vi "FRIC_navX_Internal_SPI_ProcessingLoop.vi"(7 "Device Number":T2, 11 "Rate (4Hz-200Hz)":u8=50 min=4 max=200) -> ()   [LabVIEW 2016]
doc: "This navX VI handles the reading/writing for the navX. All of the good stuff is in here.\nTHIS VI SHOULD NOT BE CALLED BY THE USER!"
uses:
  <vilib>/Rock Robotics/SystemInterfaces/spilib/spi_bus.ctl
  _TypeDefs/FRIC_navX_DeviceNumbersTypeDef.ctl
  _TypeDefs/FRIC_navX_I2C Process Loop TypeDef.ctl
  _TypeDefs/FRIC_navX_ProcessingLoopStatesTypeDef_I2C.ctl
  _TypeDefs/Z900_navX_DeviceTypeDef.ctl
  _TypeDefs/Z900_navX_ProtocolTypeDef.ctl
  _TypeDefs/Z900_navX_NotifyPacketTypeDef.ctl
  _TypeDefs/Z900_navX_ActionTypeDef.ctl
  _TypeDefs/Z900_navX_SerialStreamTypeDef.ctl
  <vilib>/Rock Robotics/SystemInterfaces/i2clib/i2c_bus.ctl
  _TypeDefs/Z900_navX_IntegrationControlRegisters.ctl
  <vilib>/Rock Robotics/WPI/SPI/WPI_SPIDevRef.ctl
  <vilib>/Rock Robotics/WPI/SerialPort/WPI_SerialPort.ctl
  <vilib>/Rock Robotics/WPI/SerialPort/WPI_SerialPortRef.ctl
  <vilib>/Platform/TimedLoop/XDataNode/timing_clust.ctl
  <vilib>/Platform/TimedLoop/XDataNode/nitl_modes.ctl
  <vilib>/Platform/TimedLoop/XDataNode/wakeup.ctl
  _TypeDefs/Flags/Z900_navX_Flags_CapabilityTypeDef.ctl
  _TypeDefs/Z900_navX_DeviceRegisters.ctl
  _Util/Z900_navX_Util_LittleEndian_to_BigEndian.vi
  <vilib>/Rock Robotics/SystemInterfaces/Utilities/FPGA_UtilitiesRead LocalTime.vi
  <vilib>/Platform/TimedLoop/XDataNode/XDataNode.xnode
  <vilib>/Platform/TimedLoop/XDataNode/XDNodeRunTimeDep.lvlib
  <vilib>/ptbypt/NI_PtbyPt.lvlib
panel:
  in  "Tab Control":enum32{"Page 1", "Page 2"}(tab)
  in  "Halt":bool
  out "Connected":bool
  in  "SPI Bus":T1=enum."SPI MXP"
  in  "Clock Rate (Hz)":dbl=2000000.0 format="%_6f"
  out "error":errorcluster
  out "Delay":dbl
  out "Loop Time":dbl format="%0.2f"
  out "Loop dt":i64
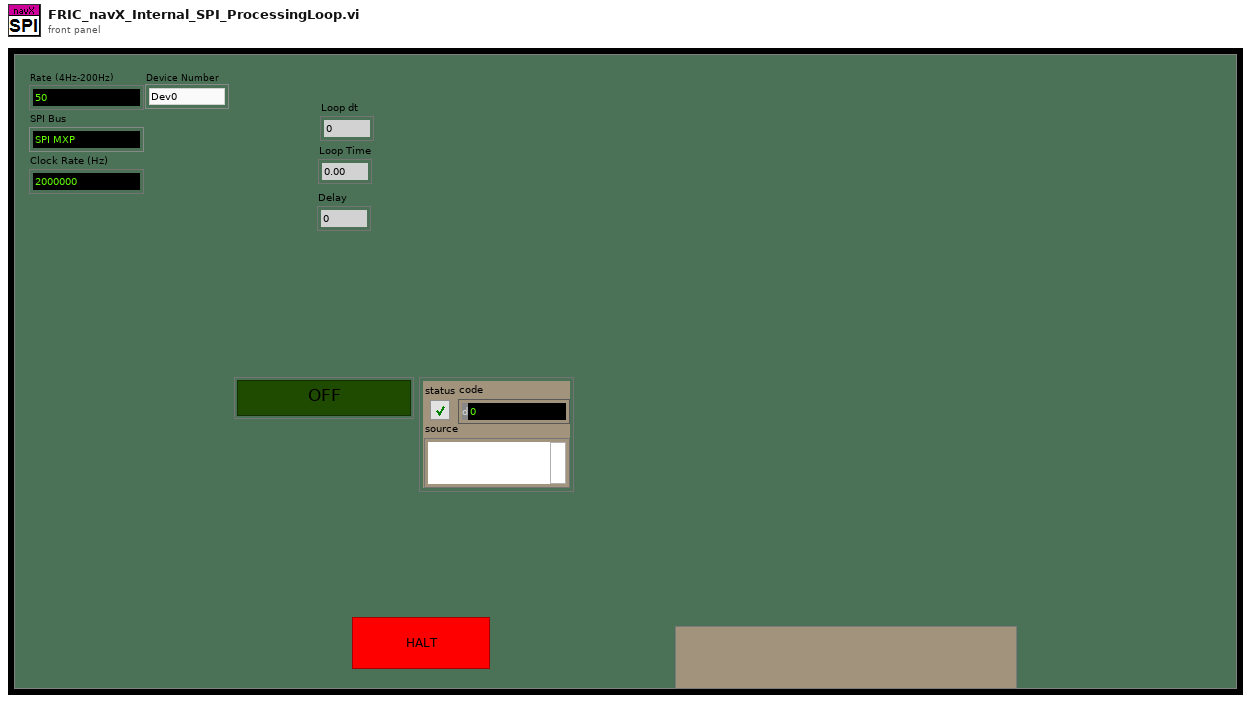
[diagram p1: front panel]
types:
  T1 = typedef "spi_bus.ctl" = enum16{"SPI On-Board, CS0", "SPI On-Board, CS1", "SPI On-Board, CS2", "SPI On-Board, CS3", "SPI MXP", "Invalid"}
  T2 = typedef "FRIC_navX_DeviceNumbersTypeDef.ctl" = enum16{"Dev0", "Dev1", "Dev2", "Dev3", "Dev4", "Dev5", "Dev6", "Dev7", "Dev8", "Dev9", "Dev10"}
  T3 = typedef "FRIC_navX_I2C Process Loop TypeDef.ctl" = cluster{"State Array":T4[], "error":errorcluster, "FPGA Cluster":cluster{"Last Valid FPGA Time":dbl, "Error Count":i32, "Initialized":bool}, "Device Info":T5, "I2CDevRef":cluster{"DevStatus":errorcluster, "Device Address":u8, "Handle":i32, "I2C Bus":T7}, "Registry":u8[], "Command Array":T8[], "Connected?":bool, "navX Device Memory Size":i32, "notification":T9, "Memory Size Set":bool, "SPIDevRef":T12, "navX Serial Open":cluster{"Stream Type":T11, "Serial Port":T13}, "SerialPortRef":T14, "Serial Read Buffer":string, "Serial Write Buffer":string[], "Device Number":T2, "navX SPI Open":cluster{"SPI Bus":T1, "Clock Rate (Hz)":dbl}, "Loop dt":i64, "current time":timestamp, "Loop Time":i64}
  T4 = typedef "FRIC_navX_ProcessingLoopStatesTypeDef_I2C.ctl" = enum16{"Process", "INI", "Check Packets Valid", "Close", "Flush Serial", "Generate Command", "Last Packet Valid", "Open", "Read", "Reset Serial", "Set Termination Char", "Update AE", "Wait", "Write", "Exit"}
  T5 = typedef "Z900_navX_DeviceTypeDef.ctl" = cluster{"Interface":cluster{"Protocol":T6, "Update Rate (4Hz-200Hz)":u8, "navX Open TypeDef":variant}, "Notify Packet":refnum<notifier>, "Loop VI Refnum":refnum<vi>, "Ready to Close Occurrence Refnum":refnum<k4>, "Name":string}
  T6 = typedef "Z900_navX_ProtocolTypeDef.ctl" = enum16{"SERIAL", "I2C", "SPI"}
  T7 = typedef "i2c_bus.ctl" = enum16{"I2C On-Board", "I2C MXP", "Invalid"}
  T8 = typedef "Z900_navX_IntegrationControlRegisters.ctl" = u8
  T9 = typedef "Z900_navX_NotifyPacketTypeDef.ctl" = cluster{"navX Action":T10, "Data":variant, "Stream Type":T11, "Device Number":T2}
  T10 = typedef "Z900_navX_ActionTypeDef.ctl" = enum16{"None", "Halt", "Normal Read", "Update Serial Protocol", "Update Rate Htz", "Zero-Yaw", "Zero-Displacement", "Zero-Velocity"}
  T11 = typedef "Z900_navX_SerialStreamTypeDef.ctl" = enum16{"YRPH", "Quaterinons", "Gyro/Raw", "AHRS", "AHRSAndPositioning", "AHRSAndPOSTime"}
  T12 = typedef "WPI_SPIDevRef.ctl" = cluster{"DevStatus":errorcluster, "Handle":i32, "SPI Bus":T1}
  T13 = typedef "WPI_SerialPort.ctl" = enum16{"Onboard RS-232", "MXP TTL", "USB 1", "USB 2"}
  T14 = typedef "WPI_SerialPortRef.ctl" = cluster{"DevStatus":errorcluster, "Serial Port Name":refnum<visa-resource-name>}
  T15 = typedef "XDNodeRunTimeDep.lvlib/timing_clust.ctl" = cluster{"Expected End [f-1]":u64, "Actual End [f-1]":u64, "Finished Late? [f-1]":bool, "Expected End [i-1]":u64, "Actual End [i-1]":u64, "Finished Late? [i-1]":bool, "Expected Start [i]":u64, "Actual Start [i]":u64, "Expected Start [f]":u64, "Actual Start [f]":u64, "Source Name":string, "Structure Name":string, "Period":i64, "Deadline":i64, "Offset":i64, "Start":i64, "Priority":i32, "Timeout":i32, "Mode":T16, "Wakeup Reason":T17, "Error":errorcluster, "Source Type":string, "Secondary Source Type":string, "Global End Time":u64, "Global Start Time":u64, "Frame Duration":u64, "Iteration Duration":u64, "Assigned CPU":i32, "I/O Scan Engine Mode":u32}
  T16 = typedef "XDNodeRunTimeDep.lvlib/nitl_modes.ctl" = enum32{"No Change", "Process missed periods, maintain original phase", "Discard missed periods, maintain original phase", "Process missed periods, ignore original phase", "Discard missed periods, ignore original phase"}
  T17 = typedef "XDNodeRunTimeDep.lvlib/wakeup.ctl" = enum32{"Normal", "Aborted", "Asynchronous wakeup", "Timing source error", "Timed loop error", "Timeout"}
  T18 = typedef "Z900_navX_DeviceRegisters.ctl" = u8
  T19 = typedef "Z900_navX_Flags_CapabilityTypeDef.ctl" = u16
  T20 = cluster{"Last Valid FPGA Time":dbl, "Error Count":i32, "Initialized":bool}
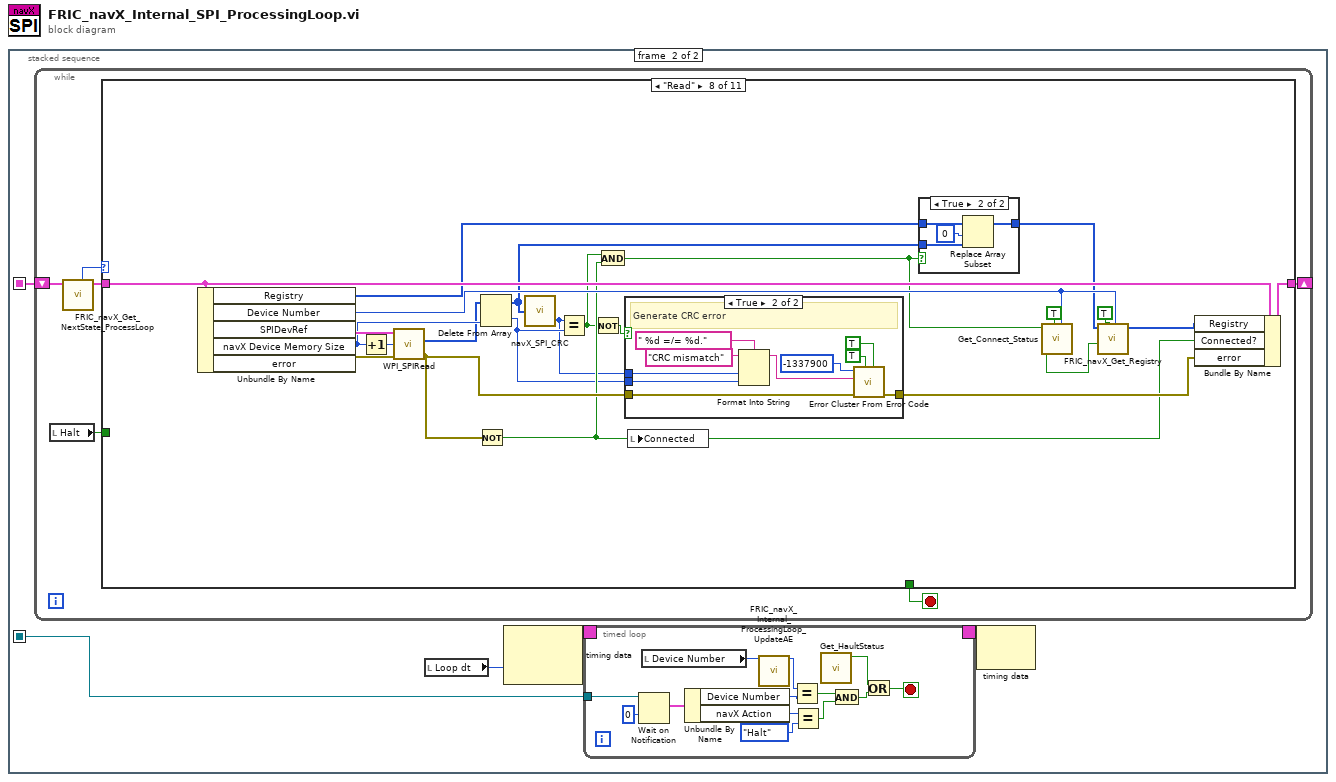
[diagram p0: block diagram]
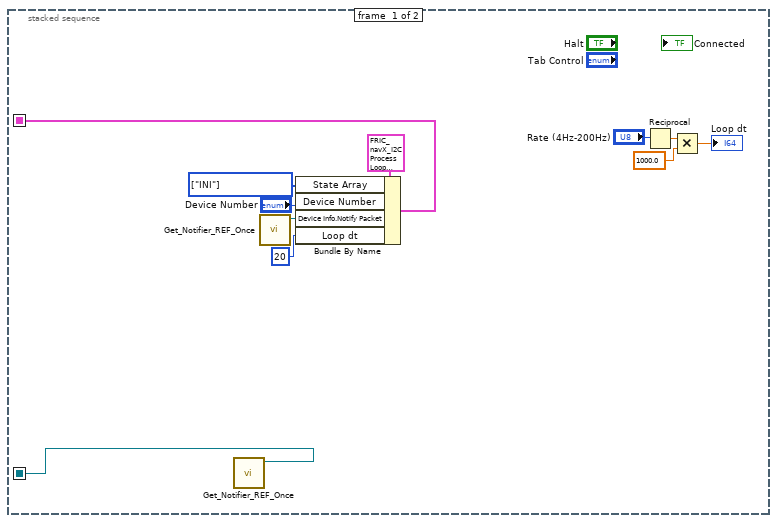
[diagram p2: hidden frame]
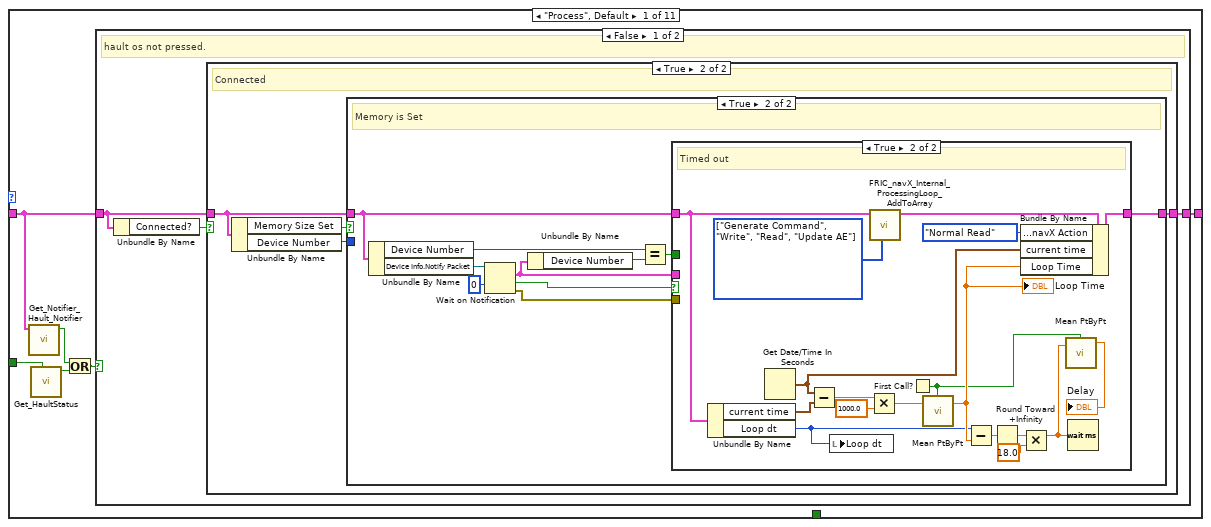
[diagram p3: hidden frame]
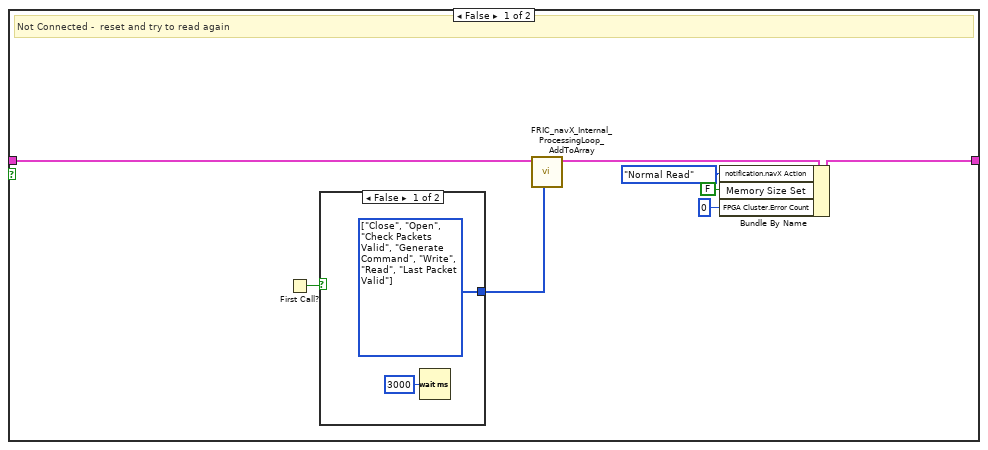
[diagram p4: hidden frame]
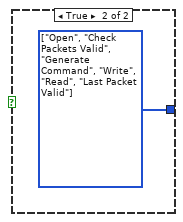
[diagram p5: hidden frame]
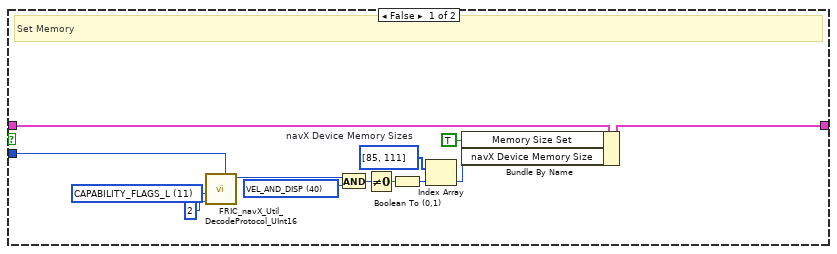
[diagram p6: hidden frame]
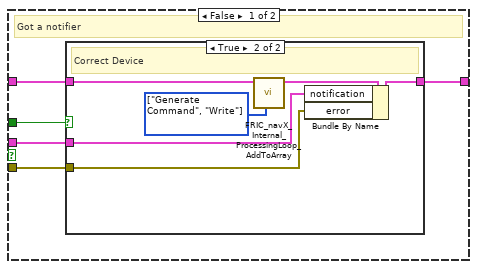
[diagram p7: hidden frame]
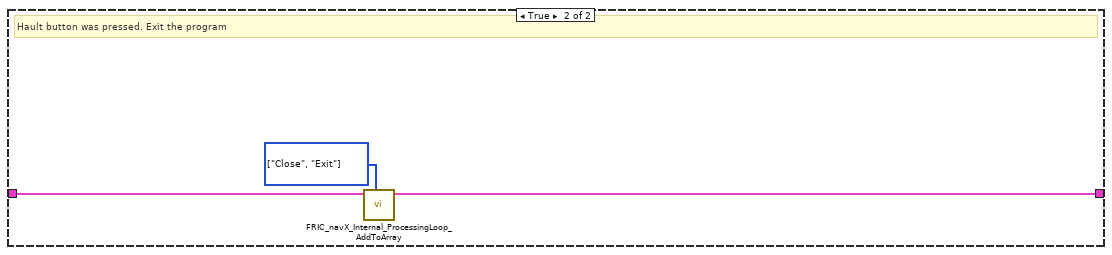
[diagram p9: hidden frame]
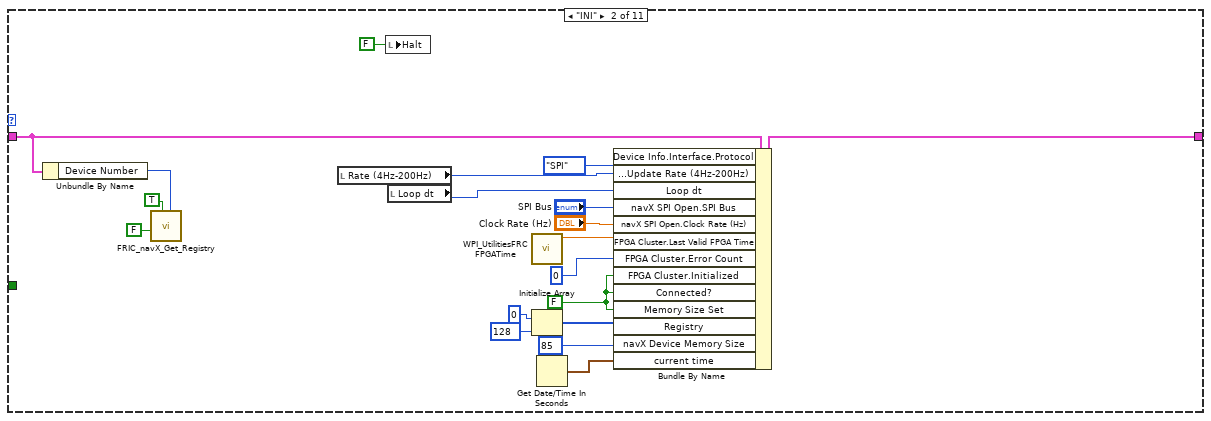
[diagram p10: hidden frame]
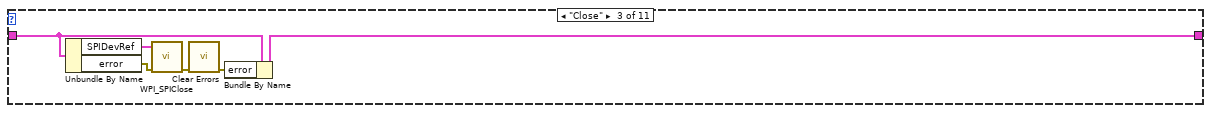
[diagram p11: hidden frame]
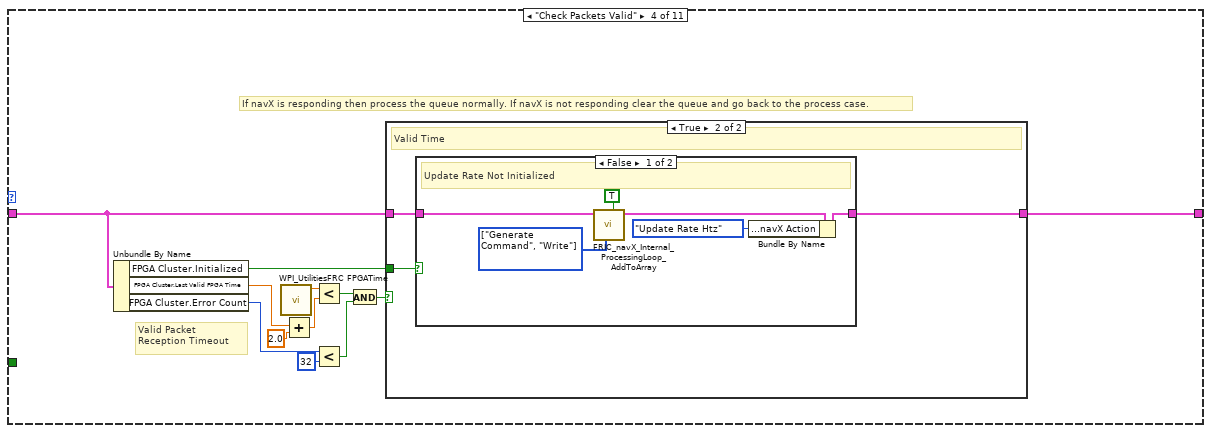
[diagram p12: hidden frame]
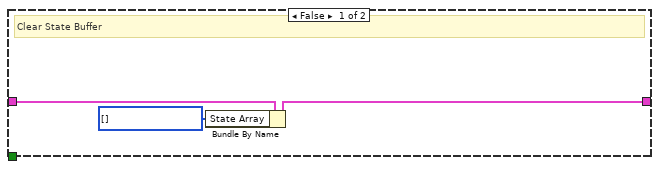
[diagram p13: hidden frame]
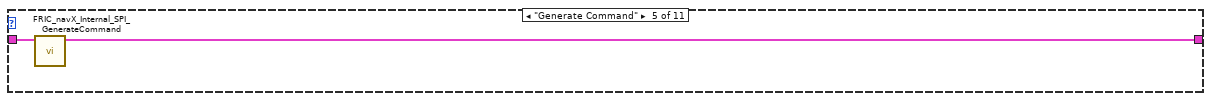
[diagram p15: hidden frame]
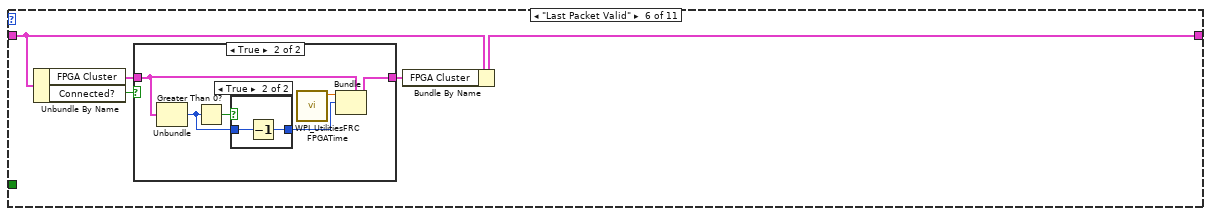
[diagram p16: hidden frame]
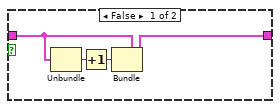
[diagram p17: hidden frame]
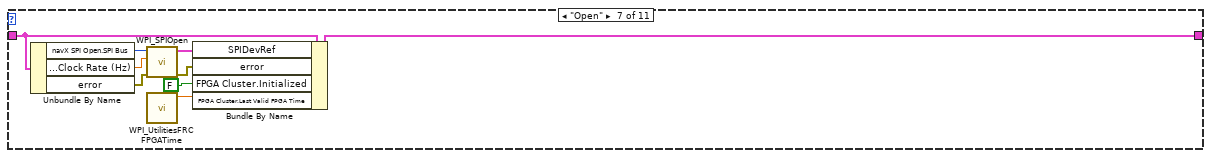
[diagram p19: hidden frame]
diagram:
  n1 = stacked-sequence {
    seq-local: [w11 _] -> [_ w16]
    seq-local: [w5 _] -> [_ w15]
    frame #0 {
      w9 = T4[] [enum."INI"] items=["Process", "INI", "Check Packets Valid", "Close", "Flush Serial", "Generate Command", "Last Packet Valid", "Open", "Read", "Reset Serial", "Set Termination Char", "Update AE", "Wait", "Write", "Exit"] ("State Array")
      n2 = call "Get_Notifier_REF_Once.vi"() -> ("notifier ref out"=w5:refnum<notifier>)  [unwired: 10 in, 1 out]
      n3 = call "Get_Notifier_REF_Once.vi"() -> ("notifier ref out"=w7:refnum<notifier>)  [unwired: 10 in, 1 out]
      n4 = Bundle By Name(cluster=T3 {"State Array"=[enum."INI", enum."Open"], "error"={"status"=FALSE, "code"=0, "source"=""}, "FPGA Cluster"={"Last Valid FPGA Time"=0.0, "Error Count"=0, "Initialized"=FALSE}, "Device Info"={"Interface"={"Protocol"=enum."SERIAL", "Update Rate (4Hz-200Hz)"=4, "navX Open TypeDef"=variant}, "Notify Packet"=refnum, "Loop VI Refnum"=refnum, "Ready to Close Occurrence Refnum"=refnum, "Name"=""}, "I2CDevRef"={"DevStatus"={"status"=FALSE, "code"=0, "source"=""}, "Device Address"=0, "Handle"=0, "I2C Bus"=enum."Invalid"}, "Registry"=[], "Command Array"=[214, 32], "Connected?"=FALSE, "navX Device Memory Size"=85, "notification"={"navX Action"=enum."None", "Data"=variant, "Stream Type"=enum."YRPH", "Device Number"=enum."Dev0"}, "Memory Size Set"=FALSE, "SPIDevRef"={"DevStatus"={"status"=FALSE, "code"=0, "source"=""}, "Handle"=0, "SPI Bus"=enum."SPI On-Board, CS0"}, "navX Serial Open"={"Stream Type"=enum."YRPH", "Serial Port"=enum."Onboard RS-232"}, "SerialPortRef"={"DevStatus"={"status"=FALSE, "code"=0, "source"=""}, "Serial Port Name"=""}, "Serial Read Buffer"="", "Serial Write Buffer"=[], "Device Number"=enum."Dev0", "navX SPI Open"={"SPI Bus"=enum."SPI MXP", "Clock Rate (Hz)"=500000.0}, "Loop dt"=0, "current time"=timestamp(0 s since 1904-01-01), "Loop Time"=0} ("I2C Process Loop TypeDef"), "State Array"=w9, "Device Number"="Device Number", "Device Info.Notify Packet"=w7, "Loop dt"=i64 20) -> (w11:T3)
      n5 = Reciprocal(x="Rate (4Hz-200Hz)") -> (1/x=w2:dbl)
      n6 = Multiply(x=w2, y=1000.0) -> (x*y=→"Loop dt":dbl)
    }
    frame #1 {
      n7 = while {
        shift-right: [w36] -> _
        shift-left: w16 -> [w39]
        stop <- w40 stop-if-true
        n8 = local read "Halt"() -> (w35:bool)
        n9 = call "FRIC_navX_Get_NextState_ProcessLoop.vi"("I2C Process Loop TypeDef (in)"=w39) -> ("I2C Process Loop TypeDef (out)"=w38:T3, "Current State"=w37:T4)  [unwired: 9 in]
        n10 = case shown="\"Read\"" w37 {
          tunnel: [_ _ _ _ _ _ _ _ _ w245 _] -> w40
          tunnel: w38 -> [w45 w127 w145 w149 w172 w176 w199 w221 w243 w247 w255]
          tunnel: [w46 w133 w144 w150 w171 w175 w198 w220 w244 w247 w255] -> w36
          tunnel: w35 -> [w43 _ _ _ _ _ _ _ _ _ _]
          frame "Process", Default {
            n11 = call "Get_Notifier_Hault_Notifier.vi"("Process Loop TypeDef (in)"=w45) -> ("Hault Notifier"=w41:bool)  [unwired: 10 in]
            n12 = call "Get_HaultStatus.vi"("Update"=w43) -> ("Hault"=w42:bool)  [unwired: 10 in]
            n13 = Or(x=w41, y=w42) -> (x .or. y?=w44:bool)
            n14 = case shown="False" w44 {
              tunnel: [w49 w119] -> w46
              tunnel: w45 -> [w47 w120]
              frame False {
                # "hault os not pressed."
                n15 = Unbundle By Name(w47) -> ("Connected?"=w48:bool)
                n16 = case shown="True" w48 {
                  tunnel: w47 -> [w57 w63]
                  tunnel: [w54 w64] -> w49
                  frame False {
                    # "Not Connected -  reset and try to read again"
                    n17 = First Call?() -> (First Call?: T/F=w50:bool)
                    n18 = case shown="False" w50 {
                      tunnel: [w59 w60] -> w56
                      frame False {
                        w59 = T4[] [enum."Close", enum."Open", enum."Check Packets Valid", enum."Generate Command", enum."Write", enum."Read", enum."Last Packet Valid"] items=["Process", "INI", "Check Packets Valid", "Close", "Flush Serial", "Generate Command", "Last Packet Valid", "Open", "Read", "Reset Serial", "Set Termination Char", "Update AE", "Wait", "Write", "Exit"]
                        n19 = Wait (ms)(milliseconds to wait=u32 3000) -> ()  [unwired: 1 out]
                      }
                      frame True {
                        w60 = T4[] [enum."Open", enum."Check Packets Valid", enum."Generate Command", enum."Write", enum."Read", enum."Last Packet Valid"] items=["Process", "INI", "Check Packets Valid", "Close", "Flush Serial", "Generate Command", "Last Packet Valid", "Open", "Read", "Reset Serial", "Set Termination Char", "Update AE", "Wait", "Write", "Exit"]
                      }
                    }
                    n20 = call "FRIC_navX_Internal_ProcessingLoop_AddToArray.vi"("States Array"=w56, "I2C Process Loop TypeDef (in)"=w57) -> ("I2C Process Loop TypeDef (out)"=w55:T3)  [unwired: 9 in]
                    n21 = Bundle By Name(cluster=w55, "notification.navX Action"=Z900_navX_ActionTypeDef."Normal Read", "Memory Size Set"=FALSE, "FPGA Cluster.Error Count"=0) -> (w54:T3)
                  }
                  frame True {
                    # "Connected"
                    n22 = Unbundle By Name(w63) -> ("Memory Size Set"=w62:bool, "Device Number"=w61:T2)
                    n23 = case shown="True" w62 {
                      tunnel: [w76 w85] -> w64
                      tunnel: w63 -> [w77 w83]
                      tunnel: w61 -> [w65 _]
                      frame False {
                        w75 = T18 11 items=["WHOAMI"=0, "HW_REV"=1, "FW_VER_MAJOR"=2, "FW_VER_MINOR"=3, "UPDATE_RATE_HZ"=4, "ACCEL_FSR_G"=5, "GYRO_FSR_DPS"=6, "OP_STATUS"=8, "CAL_STATUS"=9, "SELFTEST_STATUS"=10, "CAPABILITY_FLAGS_L"=11, "CAPABILITY_FLAGS_H"=12, "SENSOR_STATUS"=16, "TIMESTAMP"=18, "YAW"=22, "ROLL"=24, "PITCH"=26, "HEADING"=28, "FUSED_HEADING"=30, "ALTITUDE_I"=32, "ALTITUDE_D"=34, "LINERA_ACC_X"=36, "LINERA_ACC_Y"=38, "LINERA_ACC_Z"=40, "QUAT_W"=42, "QUAT_X"=44, "QUAT_Y"=46, "QUAT_Z"=48, "MPU_TEMP_C"=50, "GYRO_X"=52, "GYRO_Y"=54, "GYRO_Z"=56, "ACC_X"=58, "ACC_Y"=60, "ACC_Z"=62, "MAG_X"=64, "MAG_Y"=66, "MAG_Z"=68, "PRESSURE_I"=70, "PRESSURE_D"=72, "PRESSURE_TEMP"=74, "YAW_OFFSET"=76, "QUAT_OFFSET_W"=78, "QUAT_OFFSET_X"=80, "QUAT_OFFSET_Y"=82, "QUAT_OFFSET_Z"=84, "INTEGRATION_CONTROL"=86, "VELOCITY_X"=88, "VELOCITY_Y"=92, "VELOCITY_Z"=96, "DISPLACMENT_X"=100, "DISPLACMENT_Y"=104, "DISPLACEMENT_Z"=108] ("Device Register")
                        w70 = T19 40 items=["OMNIMOUNT"=4, "OMNIMOUNT_CONFIG_MASK"=38, "VEL_AND_DISP"=40, "YAW_RESET"=80] ("Capability Flag")
                        w71 = i32[] [85, 111]  # navX Device Memory Sizes
                        # "Set Memory"
                        n24 = call "FRIC_navX_Util_DecodeProtocol_UInt16.vi"("Device Number"=w65, "length"=2, "Device Register"=w75) -> ("Value"=w68:u16)  [unwired: 8 in]
                        n25 = And(x=w68, y=w70) -> (x .and. y?=w69:T19)
                        n26 = Not Equal To 0?(x=w69) -> (x != 0?=w72:bool)
                        n27 = Boolean To (0,1)(Boolean=w72) -> (0, 1=w73:i16)
                        n28 = Index Array(array=w71, index=w73) -> (element=w66:i32)
                        n29 = Bundle By Name(cluster=w77, "Memory Size Set"=TRUE, "navX Device Memory Size"=w66) -> (w76:T3)
                      }
                      frame True {
                        # "Memory is Set"
                        n30 = Unbundle By Name(w83) -> ("Device Number"=w80:T2, "Device Info.Notify Packet"=w87:refnum<notifier>)
                        n31 = Wait on Notification(notifier=w87, timeout in ms (-1)=0) -> (notification=w81:T9, timed out?=w82:bool, error out=w84:errorcluster)  [unwired: 2 in, 1 out]
                        n32 = Unbundle By Name(w81) -> ("Device Number"=w79:T2)
                        n33 = Equal?(x=w80, y=w79) -> (x = y?=w78:bool)
                        n34 = case shown="True" w82 {
                          tunnel: w83 -> [w92 w113]
                          tunnel: [w91 w115] -> w85
                          tunnel: w81 -> [w90 _]
                          tunnel: w84 -> [w89 _]
                          tunnel: w78 -> [w88 _]
                          frame False {
                            # "Got a notifier"
                            n35 = case shown="True" w88 {
                              tunnel: w92 -> [w93 w99]
                              tunnel: [w93 w98] -> w91
                              tunnel: w90 -> [_ w97]
                              tunnel: w89 -> [_ w94]
                              frame False {
                              }
                              frame True {
                                w95 = T4[] [enum."Generate Command", enum."Write"] items=["Process", "INI", "Check Packets Valid", "Close", "Flush Serial", "Generate Command", "Last Packet Valid", "Open", "Read", "Reset Serial", "Set Termination Char", "Update AE", "Wait", "Write", "Exit"] ("States Array")
                                # "Correct Device"
                                n36 = call "FRIC_navX_Internal_ProcessingLoop_AddToArray.vi"("States Array"=w95, "I2C Process Loop TypeDef (in)"=w99) -> ("I2C Process Loop TypeDef (out)"=w96:T3)  [unwired: 9 in]
                                n37 = Bundle By Name(cluster=w96, "notification"=w97, "error"=w94) -> (w98:T3)
                              }
                            }
                          }
                          frame True {
                            w117 = T4[] [enum."Generate Command", enum."Write", enum."Read", enum."Update AE"] items=["Process", "INI", "Check Packets Valid", "Close", "Flush Serial", "Generate Command", "Last Packet Valid", "Open", "Read", "Reset Serial", "Set Termination Char", "Update AE", "Wait", "Write", "Exit"]
                            # "Timed out"
                            n38 = Unbundle By Name(w113) -> ("current time"=w112:timestamp, "Loop dt"=w100:i64)
                            n39 = Get Date/Time In Seconds() -> (seconds since 1Jan1904=w111:timestamp)
                            n40 = Subtract(x=w111, y=w112) -> (x-y=w110:dbl)
                            n41 = local write "Loop dt"(w100) -> ()
                            n42 = Multiply(x=w110, y=1000.0) -> (x*y=w107:dbl)
                            n43 = call "FRIC_navX_Internal_ProcessingLoop_AddToArray.vi"("States Array"=w117, "I2C Process Loop TypeDef (in)"=w113) -> ("I2C Process Loop TypeDef (out)"=w116:T3)  [unwired: 9 in]
                            n44 = First Call?() -> (First Call?: T/F=w101:bool)
                            n45 = call <vilib>:"Mean PtByPt.vi"("x"=w107, "initialize"=w101) -> ("mean"=w106:dbl)  [unwired: 2 in, 1 out]
                            "Loop Time" <- w106
                            n46 = Subtract(x=w100, y=w106) -> (x-y=w108:dbl)
                            n47 = Round Toward +Infinity(x=w108) -> (ceil(x): smallest int >= x=w104:dbl)
                            n48 = Bundle By Name(cluster=w116, "notification.navX Action"=Z900_navX_ActionTypeDef."Normal Read", "current time"=w111, "Loop Time"=w106) -> (w115:T3)
                            n49 = Multiply(x=w104, y=18.0) -> (x*y=w103:dbl)
                            n50 = call <vilib>:"Mean PtByPt.vi"("x"=w103, "initialize"=w101) -> ("mean"=→"Delay":dbl)  [unwired: 2 in, 1 out]
                            n51 = Wait (ms)(milliseconds to wait=w103) -> ()  [unwired: 1 out]
                          }
                        }
                      }
                    }
                  }
                }
              }
              frame True {
                w118 = T4[] [enum."Close", enum."Exit"] items=["Process", "INI", "Check Packets Valid", "Close", "Flush Serial", "Generate Command", "Last Packet Valid", "Open", "Read", "Reset Serial", "Set Termination Char", "Update AE", "Wait", "Write", "Exit"] ("States Array")
                # "Hault button was pressed. Exit the program"
                n52 = call "FRIC_navX_Internal_ProcessingLoop_AddToArray.vi"("States Array"=w118, "I2C Process Loop TypeDef (in)"=w120) -> ("I2C Process Loop TypeDef (out)"=w119:T3)  [unwired: 9 in]
              }
            }
          }
          frame "INI" {
            w131 = FALSE ("Initialized")
            n53 = Unbundle By Name(w127) -> ("Device Number"=w126:T2)
            n54 = call "FRIC_navX_Get_Registry.vi"("Device Number"=w126, "Update"=TRUE, "Connected?"=FALSE) -> ()  [unwired: 7 in, 2 out]
            n55 = local read "Rate (4Hz-200Hz)"() -> (w122:u8)
            n56 = local write "Halt"(FALSE ("Halt")) -> ()
            n57 = local read "Loop dt"() -> (w121:i64)
            n58 = call <vilib>:"WPI_UtilitiesFRC FPGATime.vi"() -> ("FPGA Time"=w135:dbl)  [unwired: 10 in, 1 out]
            n59 = Initialize Array(u8 0 ("Received Data"), 128 ("hex")) -> (w129:u8[])
            n60 = Get Date/Time In Seconds() -> (seconds since 1Jan1904=w123:timestamp)
            n61 = Bundle By Name(cluster=w127, "Device Info.Interface.Protocol"=Z900_navX_ProtocolTypeDef."SPI" ("Protocol"), "Device Info.Interface.Update Rate (4Hz-200Hz)"=w122, "Loop dt"=w121, "navX SPI Open.SPI Bus"="SPI Bus", "navX SPI Open.Clock Rate (Hz)"="Clock Rate (Hz)", "FPGA Cluster.Last Valid FPGA Time"=w135, "FPGA Cluster.Error Count"=0 ("Error Count"), "FPGA Cluster.Initialized"=w131, "Connected?"=w131, "Memory Size Set"=w131, "Registry"=w129, "navX Device Memory Size"=85 ("hex"), "current time"=w123) -> (w133:T3)
          }
          frame "Close" {
            n62 = Unbundle By Name(w145) -> ("SPIDevRef"=w143:T12, "error"=w142:errorcluster)
            n63 = call <vilib>:"WPI_SPIClose.vi"("error in (no error)"=w142, "SPIDevRef"=w143) -> ("error out"=w141:errorcluster)  [unwired: 9 in]
            n64 = call <vilib>:"Clear Errors.vi"("error in (no error)"=w141) -> ("error out"=w140:errorcluster)  [unwired: 5 in, 1 out]
            n65 = Bundle By Name(cluster=w145, "error"=w140) -> (w144:T3)
          }
          frame "Check Packets Valid" {
            # "If navX is responding then process the queue normally. If navX is not responding clear the queue and go back to the process case."
            # "Valid Packet Reception Timeout"
            n66 = Unbundle By Name(w149) -> ("FPGA Cluster.Initialized"=w147:bool, "FPGA Cluster.Last Valid FPGA Time"=w148:dbl, "FPGA Cluster.Error Count"=w146:i32)
            n67 = call <vilib>:"WPI_UtilitiesFRC FPGATime.vi"() -> ("FPGA Time"=w155:dbl)  [unwired: 10 in, 1 out]
            n68 = Add(x=w148, y=2.0) -> (x+y=w156:dbl)
            n69 = Less?(x=w155, y=w156) -> (x < y?=w153:bool)
            n70 = Less?(x=w146, y=32) -> (x < y?=w152:bool)
            n71 = And(x=w153, y=w152) -> (x .and. y?=w151:bool)
            n72 = case shown="True" w151 {
              tunnel: w149 -> [w160 w163]
              tunnel: [w159 w162] -> w150
              tunnel: w147 -> [_ w161]
              frame False {
                w158 = T4[] [] items=["Process", "INI", "Check Packets Valid", "Close", "Flush Serial", "Generate Command", "Last Packet Valid", "Open", "Read", "Reset Serial", "Set Termination Char", "Update AE", "Wait", "Write", "Exit"] ("f")
                # "Clear State Buffer"
                n73 = Bundle By Name(cluster=w160, "State Array"=w158) -> (w159:T3)
              }
              frame True {
                # "Valid Time"
                n74 = case shown="False" w161 {
                  tunnel: w163 -> [w168 w170]
                  tunnel: [w166 w170] -> w162
                  frame False {
                    w164 = T4[] [enum."Generate Command", enum."Write"] items=["Process", "INI", "Check Packets Valid", "Close", "Flush Serial", "Generate Command", "Last Packet Valid", "Open", "Read", "Reset Serial", "Set Termination Char", "Update AE", "Wait", "Write", "Exit"] ("f")
                    # "Update Rate Not Initialized"
                    n75 = call "FRIC_navX_Internal_ProcessingLoop_AddToArray.vi"("Add to beginning"=TRUE, "States Array"=w164, "I2C Process Loop TypeDef (in)"=w168) -> ("I2C Process Loop TypeDef (out)"=w167:T3)  [unwired: 8 in]
                    n76 = Bundle By Name(cluster=w167, "notification.navX Action"=Z900_navX_ActionTypeDef."Update Rate Htz") -> (w166:T3)
                  }
                  frame True {
                    # "Update Rate is Initialized"
                  }
                }
              }
            }
          }
          frame "Generate Command" {
            n77 = call "FRIC_navX_Internal_SPI_GenerateCommand.vi"("I2C Process Loop TypeDef (in)"=w172) -> ("I2C Process Loop TypeDef (out)"=w171:T3)  [unwired: 10 in]
          }
          frame "Last Packet Valid" {
            n78 = Unbundle By Name(w176) -> ("FPGA Cluster"=w177:T20, "Connected?"=w173:bool)
            n79 = case shown="True" w173 {
              tunnel: [w180 w187] -> w174
              tunnel: w177 -> [w179 w183]
              frame False {
                n80 = Unbundle(w179) -> ("Error Count"=w178:i32)  [unwired: 2 out]
                n81 = Increment(x=w178) -> (x+1=w181:i32)
                n82 = Bundle(cluster=w179, "Error Count"=w181) -> (w180:T20)  [unwired: 2 in]
              }
              frame True {
                n83 = Unbundle(w183) -> ("Error Count"=w182:i32)  [unwired: 2 out]
                n84 = Greater Than 0?(x=w182) -> (x > 0?=w185:bool)
                n85 = case shown="True" w185 {
                  tunnel: [w188 w190] -> w184
                  tunnel: w182 -> [w188 w189]
                  frame False {
                  }
                  frame True {
                    n86 = Decrement(x=w189) -> (x-1=w190:i32)
                  }
                }
                n87 = call <vilib>:"WPI_UtilitiesFRC FPGATime.vi"() -> ("FPGA Time"=w186:dbl)  [unwired: 10 in, 1 out]
                n88 = Bundle(cluster=w183, "Last Valid FPGA Time"=w186, "Error Count"=w184) -> (w187:T20)  [unwired: 1 in]
              }
            }
            n89 = Bundle By Name(cluster=w176, "FPGA Cluster"=w174) -> (w175:T3)
          }
          frame "Open" {
            n90 = Unbundle By Name(w199) -> ("navX SPI Open.SPI Bus"=w192:T1, "navX SPI Open.Clock Rate (Hz)"=w191:dbl, "error"=w193:errorcluster)
            n91 = call <vilib>:"WPI_SPIOpen.vi"("error in"=w193, "Clock Rate (Hz)"=w191, "SPI Bus"=w192) -> ("error out"=w195:errorcluster, "SPIDevRef"=w196:T12)  [unwired: 7 in]
            n92 = call <vilib>:"WPI_UtilitiesFRC FPGATime.vi"() -> ("FPGA Time"=w194:dbl)  [unwired: 10 in, 1 out]
            n93 = Bundle By Name(cluster=w199, "SPIDevRef"=w196, "error"=w195, "FPGA Cluster.Initialized"=FALSE ("Initialized"), "FPGA Cluster.Last Valid FPGA Time"=w194) -> (w198:T3)
          }
          frame "Read" {
            n94 = Unbundle By Name(w221) -> ("Registry"=w218:u8[], "Device Number"=w212:T2, "SPIDevRef"=w217:T12, "navX Device Memory Size"=w214:i32, "error"=w216:errorcluster)
            n95 = Increment(x=w214) -> (x+1=w213:i32)
            n96 = call <vilib>:"WPI_SPIRead.vi"("error in (no error)"=w216, "Num to Read"=w213, "SPIDevRef"=w217) -> ("error out"=w210:errorcluster, "Received Data"=w206:u8[])  [unwired: 6 in, 1 out]
            n97 = Not(x=w210) -> (.not. x?=w209:bool)
            n98 = Delete From Array(array=w206, index=w214) -> (deleted portion=w204:u8, array with subset deleted=w202:u8[])  [unwired: 1 in]
            n99 = call "navX_SPI_CRC.vi"("Message"=w202) -> ("CRC"=w201:u8)  [unwired: 1 out]
            n100 = Equal?(x=w201, y=w204) -> (x = y?=w205:bool)
            n101 = Not(x=w205) -> (.not. x?=w203:bool)
            n102 = And(x=w205, y=w209) -> (x .and. y?=w207:bool)
            n103 = case shown="True" w203 {
              tunnel: w201 -> [_ w230]
              tunnel: w204 -> [_ w229]
              tunnel: w210 -> [w222 w226]
              tunnel: [w222 w225] -> w215
              frame False {
              }
              frame True {
                # "Generate CRC error"
                n104 = Format Into String(format string=" %d =/= %d.", initial string="CRC mismatch", w230, w229) -> (resulting string=w227:string)  [unwired: 1 in, 1 out]
                n105 = call <vilib>:"Error Cluster From Error Code.vi"("is warning? (False)"=TRUE, "show call chain? (False)"=TRUE, "error in (no error)"=w226, "error message (\"\")"=w227, "error code (0)"=-1337900 ("code")) -> ("error out"=w225:errorcluster)  [unwired: 4 in]
              }
            }
            n106 = local write "Connected"(w209) -> ()
            n107 = case shown="True" w207 {
              tunnel: w218 -> [_ w237]
              tunnel: [w233 w236] -> w200
              tunnel: w202 -> [w233 w235]
              frame False {
              }
              frame True {
                n108 = Replace Array Subset(array=w237, new element=w235, index=u8 0 ("hex")) -> (w236:u8[])
              }
            }
            n109 = call "Get_Connect_Status.vi"("Device Number"=w212, "Update"=TRUE, "Connected"=w207) -> ()  [unwired: 8 in, 1 out]
            n110 = call "FRIC_navX_Get_Registry.vi"("Device Number"=w212, "Update"=TRUE, "Connected?"=w207, "Registry (in)"=w200) -> ("Registry (out)"=w219:u8[])  [unwired: 6 in, 1 out]
            n111 = Bundle By Name(cluster=w221, "Registry"=w219, "Connected?"=w209, "error"=w215) -> (w220:T3)
          }
          frame "Write" {
            n112 = Unbundle By Name(w243) -> ("SPIDevRef"=w242:T12, "Command Array"=w241:T8[], "I2CDevRef.DevStatus"=w240:errorcluster)
            n113 = call <vilib>:"WPI_SPIWrite.vi"("error in (no error)"=w240, "Data To Send"=w241, "SPIDevRef"=w242) -> ("error out"=w239:errorcluster, "SPIDevRef"=w238:T12)  [unwired: 6 in, 1 out]
            n114 = Bundle By Name(cluster=w243, "SPIDevRef"=w238, "error"=w239) -> (w244:T3)
          }
          frame "Exit" {
            n115 = Unbundle By Name(w247) -> ("Device Info"=w246:T5)
            n116 = in-place {
              in-place-border: [TRUE] -> w245
              in-place-border: w246 -> [w248]
              # "Set Occurence of Close"
              n117 = Unbundle By Name(w248) -> ("Ready to Close Occurrence Refnum"=w250:refnum<k4>)
              n118 = local write "Halt"(FALSE ("Halt")) -> ()
              n119 = Set Occurrence(w250) -> ()
            }
          }
          frame "Update AE" {
            n120 = Unbundle By Name(w255) -> ("Device Number"=w252:T2, "error"=w254:errorcluster)
            "error" <- w254
            n121 = call "Get_Error_Status.vi"("Device Number"=w252, "Update"=TRUE, "error in"=w254) -> ()  [unwired: 8 in, 1 out]
          }
        }
      }
      n122 = local read "Loop dt"() -> (w12:i64)
      n123 = node-c288(w12) -> (w14:T15)  [unwired: 1 in]
      n124 = timed-loop {
        timing: w14 -> [_]
        timing-out: [_] -> w13
        tunnel: w15 -> [w25]
        stop <- w17 stop-if-true
        n125 = Wait on Notification(notifier=w25, timeout in ms (-1)=0) -> (notification=w24:T9)  [unwired: 2 in, 3 out]
        n126 = local read "Device Number"() -> (w22:T2)
        n127 = Unbundle By Name(w24) -> ("Device Number"=w23:T2, "navX Action"=w27:T10)
        n128 = call "FRIC_navX_Internal_ProcessingLoop_UpdateAE.vi"("Device Number"=w22) -> ()  [unwired: 15 in]
        n129 = Equal?(x=w22, y=w23) -> (x = y?=w21:bool)
        n130 = Equal?(x=w27, y=Z900_navX_ActionTypeDef."Halt") -> (x = y?=w20:bool)
        n131 = call "Get_HaultStatus.vi"() -> ("Hault"=w19:bool)  [unwired: 11 in]
        n132 = And(x=w21, y=w20) -> (x .and. y?=w18:bool)
        n133 = Or(x=w19, y=w18) -> (x .or. y?=w17:bool)
      }
      n134 = node-c288(w13) -> ()  [unwired: 1 out]
    }
  }
